vi "Write table parameters.vi"(8 "error in (no error)":errorcluster, 10 "table parameters":T1, 11 "SP in":refnum<class "Save messages PGserver.lvclass">) -> (0 "error out":errorcluster, 3 "SP out":refnum<class "Save messages PGserver.lvclass">)   [LabVIEW 2019, in "Save messages PGserver.lvclass"]
uses:
  Save messages PGserver.lvclass
  Save messages PGserver.lvclass/Save messages PGserver.ctl
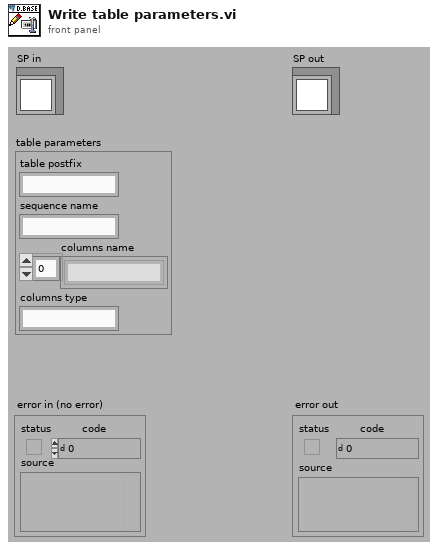
[diagram p1: front panel]
types:
  T1 = cluster{"table postfix":string, "sequence name":string, "columns name":string[], "columns type":string}
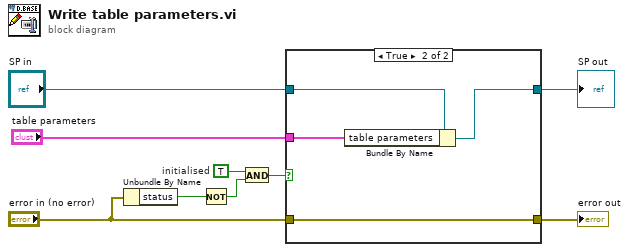
[diagram p0: block diagram]
diagram:
  w4 = TRUE  # initialised
  n1 = Unbundle By Name("error in (no error)") -> ("status"=w7:bool)
  n2 = Not(x=w7) -> (.not. x?=w6:bool)
  n3 = And(x=w4, y=w6) -> (x .and. y?=w8:bool)
  n4 = case shown="True" w8 {
    tunnel: [w11 w15] -> w9
    tunnel: "error in (no error)" -> [w11 w15]
    tunnel: "SP in" -> [w10 w14]
    tunnel: [w10 w13] -> w2
    tunnel: "table parameters" -> [_ w12]
    frame False {
    }
    frame True {
      n5 = Bundle By Name(cluster=w14, "table parameters"=w12) -> (w13:refnum<class "Save messages PGserver.lvclass">)
    }
  }
  "error out" <- w9
  "SP out" <- w2
